vi "End RPC Call.vi"(8 "error in (no error)":errorcluster, 11 "gRPCid":T1) -> (0 "error out":errorcluster)   [LabVIEW 2019, in "OCV2.lvlib" / "OCV2.lvclass"]
uses:
  OCV2.lvclass
  gRPC lvSupport/Server API/typeDefs/grpcId.ctl
  gRPC lvSupport/gprc-lvsupport.lvlib
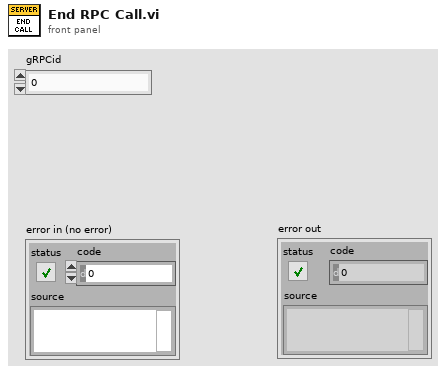
[diagram p1: front panel]
types:
  T1 = typedef "OCV2.lvlib/gprc-lvsupport.lvlib/grpcId.ctl" = u64
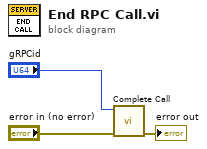
[diagram p0: block diagram]
diagram:
  n1 = call "Complete Call.vi"("gRPCid"="gRPCid", "error in (no error)"="error in (no error)") -> ("error out"=→"error out":errorcluster)  [unwired: 8 in]
